vi "Associated Research SC6540 Example - Setup the Multiplexer.vi"() -> ()   [LabVIEW 2014]
doc: "Setup the multiplexer for safety test. This VI shows the steps of how to configure the SC6540 and coordinate with the safety tester."
uses:
  <instrlib>/Associated Research SC6540/Associated Research SC6540.lvlib
panel:
  in  "Ground Bond Channel (1)":i32=5
  in  "Return Channels":i32[](array[numeric])=[2, 4, 6]
  in  "High Voltage Channels":i32[](array[numeric])=[1, 3, 5]
  in  "VISA resource name":refnum<visa-resource-name>="ASRL11::INSTR"
  # "(c) 2023 IKONIX Group.  ALL RIGHTS RESERVED."
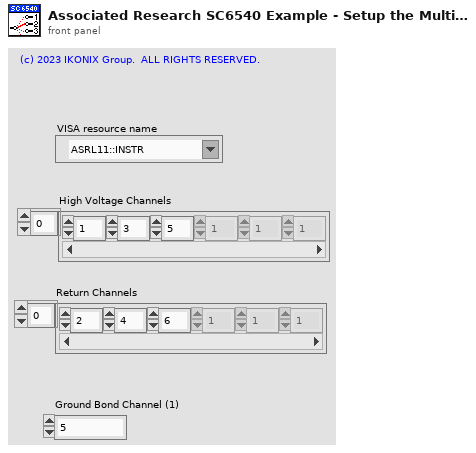
[diagram p1: front panel]
types:
  T1 = cluster{"Baud Rate":u32, "Parity":u16, "Data Bits":u16, "Stop Bits":u16, "Flow Control":u16}
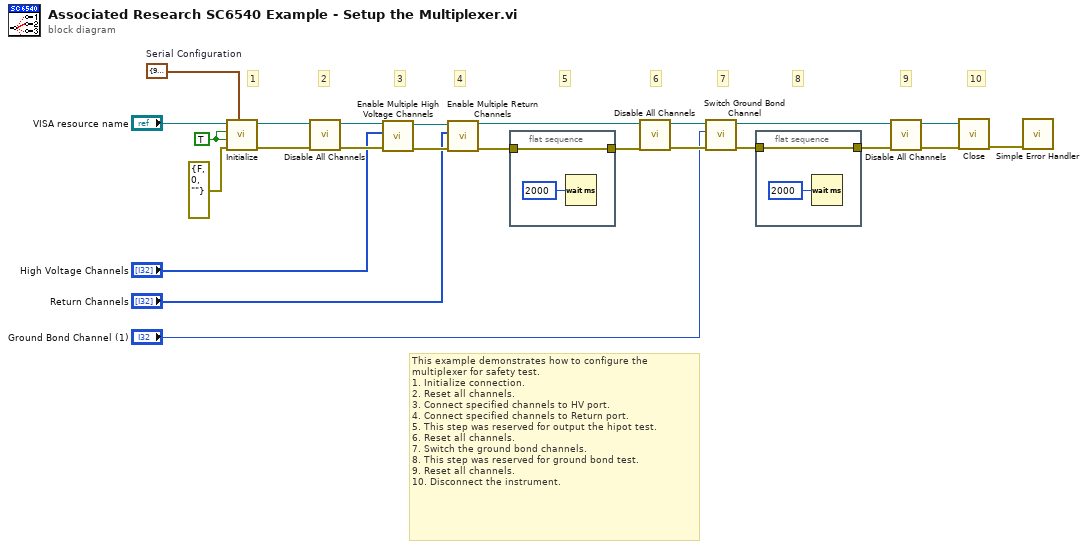
[diagram p0: block diagram]
diagram:
  w21 = T1 {"Baud Rate"=9600, "Parity"=0, "Data Bits"=8, "Stop Bits"=10, "Flow Control"=0}  # Serial Configuration
  w22 = TRUE ("ID Query (True)")
  # "This example demonstrates how to configure the multiplexer for safety test.\n1. Initialize connection.\n2. Reset all channels.\n3. Connect specified channels to HV port.\n4. Connect specified channels to Return port.\n5. This step was reserved for output the hipot test.\n6. Reset all channels.\n7. Switch the ground bond channels.\n8. This step was reserved for ground bond test.\n9. Reset all channels.\n10. Disconnect the instrument."
  # "10"
  # "9"
  # "8"
  # "7"
  # "6"
  # "5"
  # "4"
  # "3"
  # "2"
  # "1"
  n1 = call <instrlib>:"Initialize.vi"("Serial Configuration"=w21, "error in (no error)"=errorcluster {"status"=FALSE, "code"=0, "source"=""}, "Reset (True)"=w22, "ID Query (True)"=w22, "VISA resource name"="VISA resource name") -> ("error out"=w18:errorcluster, "VISA resource name out"=w19:refnum<visa-resource-name>)  [unwired: 5 in]
  n2 = call <instrlib>:"Disable All Channels.vi"("error in (no error)"=w18, "VISA resource name"=w19) -> ("error out"=w16:errorcluster, "VISA resource name out"=w17:refnum<visa-resource-name>)  [unwired: 8 in]
  n3 = call <instrlib>:"Enable Multiple High Voltage Channels.vi"("error in (no error)"=w16, "High Voltage Channels"="High Voltage Channels", "VISA resource name"=w17) -> ("error out"=w13:errorcluster, "VISA resource name out"=w14:refnum<visa-resource-name>)  [unwired: 7 in]
  n4 = call <instrlib>:"Enable Multiple Return Channels.vi"("error in (no error)"=w13, "Return Channels"="Return Channels", "VISA resource name"=w14) -> ("error out"=w11:errorcluster, "VISA resource name out"=w9:refnum<visa-resource-name>)  [unwired: 7 in]
  n5 = flat-sequence {
    tunnel: w11 -> [w25]
    tunnel: [w25] -> w10
    frame #0 {
      n6 = Wait (ms)(milliseconds to wait=u32 2000) -> ()  [unwired: 1 out]
    }
  }
  n7 = call <instrlib>:"Disable All Channels.vi"("error in (no error)"=w10, "VISA resource name"=w9) -> ("error out"=w7:errorcluster, "VISA resource name out"=w8:refnum<visa-resource-name>)  [unwired: 8 in]
  n8 = call <instrlib>:"Switch Ground Bond Channel.vi"("error in (no error)"=w7, "Channel (1)"="Ground Bond Channel (1)", "VISA resource name"=w8) -> ("error out"=w5:errorcluster, "VISA resource name out"=w3:refnum<visa-resource-name>)  [unwired: 7 in]
  n9 = flat-sequence {
    tunnel: w5 -> [w27]
    tunnel: [w27] -> w4
    frame #0 {
      n10 = Wait (ms)(milliseconds to wait=u32 2000) -> ()  [unwired: 1 out]
    }
  }
  n11 = call <instrlib>:"Disable All Channels.vi"("error in (no error)"=w4, "VISA resource name"=w3) -> ("error out"=w1:errorcluster, "VISA resource name out"=w2:refnum<visa-resource-name>)  [unwired: 8 in]
  n12 = call <instrlib>:"Close.vi"("error in (no error)"=w1, "VISA resource name"=w2) -> ("error out"=w20:errorcluster)  [unwired: 9 in]
  n13 = call <vilib>:"Simple Error Handler.vi"("error in (no error)"=w20) -> ()  [unwired: 4 in, 5 out]
